vi "appendTable.vi"(8 "error in (no error)":errorcluster, 9 "Cell.Style":refnum<class "Style.lvclass">, 10 "Table":string[][](array[string]), 11 "xwpfTable in":refnum<class "xwpfTable.lvclass">) -> (0 "error out":errorcluster, 3 "xwpfTable out":refnum<class "xwpfTable.lvclass">)   [LabVIEW 2017, in "Word_Specific.lvlib" / "xwpfTable.lvclass"]
uses:
  xwpfTable.lvclass
  Styles/Style/Style.lvclass
  xwpfTable.lvclass/xwpfTable.ctl
  C:/Users/Neo/Desktop/Dev_Tools_BR/LabVIEW_NPOI/src/lib/NPOI 2.1.1/NPOI.OOXML.dll
  lib/NPOI 2.1.1/NPOI.OOXML.dll
  xwpfParagraph/xwpfParagraph.lvclass
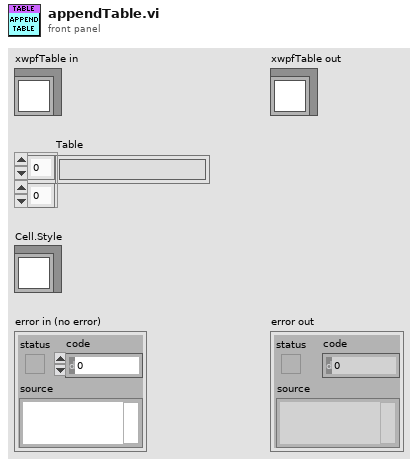
[diagram p1: front panel]
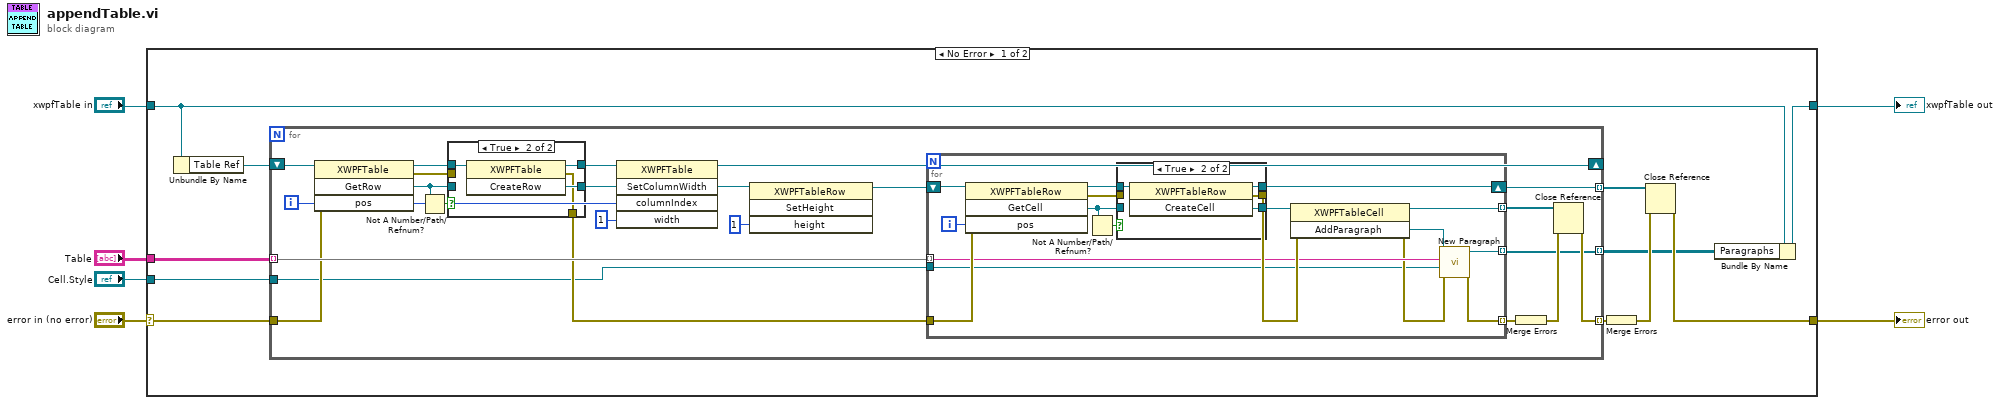
[diagram p0: block diagram]
diagram:
  n1 = case shown="No Error" "error in (no error)" {
    selector: "error in (no error)" -> [w13 w72]
    tunnel: [w12 w72] -> w5
    tunnel: [w9 w71] -> w3
    tunnel: "xwpfTable in" -> [w17 w71]
    tunnel: "Table" -> [w15 _]
    tunnel: "Cell.Style" -> [w7 _]
    frame No Error {
      n2 = Unbundle By Name(w17) -> ("Table Ref"=w16:refnum<k24>)
      n3 = for {
        shift-right: [w22] -> _
        shift-left: w16 -> [w39]
        tunnel: w15 -> [w35] mode=indexing
        tunnel: [w34] -> w14 mode=indexing
        tunnel: [w27] -> w11 mode=indexing
        tunnel: w13 -> [w30]
        tunnel: [w26] -> w8 mode=indexing
        tunnel: w7 -> [w25]
        i -> [w23]
        n4 = invoke class="XWPFTable" method="GetRow"(reference=w39, error in=w30, "pos"=w23) -> (reference out=w36:refnum<k24>, error out=w32:errorcluster, "GetRow"=w37:refnum<k24>)  [unwired: 1 in, 1 out]
        n5 = Not A Number/Path/Refnum?(number/path/refnum=w37) -> (NaN/Path/Refnum?=w38:bool)
        n6 = case shown="True" w38 {
          tunnel: w37 -> [w66 _]
          tunnel: w36 -> [w65 w70]
          tunnel: [w66 w69] -> w21
          tunnel: [w65 w68] -> w24
          tunnel: [w64 w67] -> w31
          tunnel: w32 -> [w64 _]
          frame False {
          }
          frame True {
            n7 = invoke class="XWPFTable" method="CreateRow"(reference=w70) -> (reference out=w68:refnum<k24>, error out=w67:errorcluster, "CreateRow"=w69:refnum<k24>)  [unwired: 2 in]
          }
        }
        n8 = invoke class="XWPFTable" method="SetColumnWidth"(reference=w24, "columnIndex"=w23, "width"=u64 1) -> (reference out=w22:refnum<k24>)  [unwired: 2 in, 4 out]
        n9 = invoke class="XWPFTableRow" method="SetHeight"(reference=w21, "height"=1) -> (reference out=w20:refnum<k24>)  [unwired: 2 in, 3 out]
        n10 = for {
          shift-right: [w51] -> w34
          shift-left: w20 -> [w56]
          tunnel: w35 -> [w44] mode=indexing
          tunnel: [w49] -> w33 mode=indexing
          tunnel: [w42] -> w29 mode=indexing
          tunnel: w31 -> [w48]
          tunnel: [w41] -> w26 mode=indexing
          tunnel: w25 -> [w40]
          i -> [w55]
          n11 = invoke class="XWPFTableRow" method="GetCell"(reference=w56, error in=w48, "pos"=w55) -> (reference out=w54:refnum<k24>, error out=w47:errorcluster, "GetCell"=w53:refnum<k24>)  [unwired: 1 in, 1 out]
          n12 = Not A Number/Path/Refnum?(number/path/refnum=w53) -> (NaN/Path/Refnum?=w52:bool)
          n13 = case shown="True" w52 {
            tunnel: w53 -> [w59 _]
            tunnel: w54 -> [w58 w63]
            tunnel: [w59 w62] -> w50
            tunnel: [w58 w61] -> w51
            tunnel: w47 -> [w57 _]
            tunnel: [w57 w60] -> w46
            frame False {
            }
            frame True {
              n14 = invoke class="XWPFTableRow" method="CreateCell"(reference=w63) -> (reference out=w61:refnum<k24>, error out=w60:errorcluster, "CreateCell"=w62:refnum<k24>)  [unwired: 2 in]
            }
          }
          n15 = invoke class="XWPFTableCell" method="AddParagraph"(reference=w50, error in=w46) -> (reference out=w49:refnum<k24>, error out=w43:errorcluster, "AddParagraph"=w45:refnum<k24>)  [unwired: 1 in]
          n16 = call "New Paragraph.vi"("error in (no error)"=w43, "Paragraph.Style"=w40, "Paragraph.Text"=w44, "Paragraph.Ref"=w45) -> ("error out"=w42:errorcluster, "xwpfParagraph out"=w41:refnum<class "xwpfParagraph.lvclass">)  [unwired: 6 in]
        }
        n17 = Merge Errors(w29) -> (w28:errorcluster)
        n18 = Close Reference(reference=w33, error in (no error)=w28) -> (error out=w27:errorcluster)
      }
      n19 = Merge Errors(w11) -> (w10:errorcluster)
      n20 = Close Reference(reference=w14, error in (no error)=w10) -> (error out=w12:errorcluster)
      n21 = Bundle By Name(cluster=w17, "Paragraphs"=w8) -> (w9:refnum<class "xwpfTable.lvclass">)
    }
    frame Error {
    }
  }
  "error out" <- w5
  "xwpfTable out" <- w3
